vi "MALT132 get several output.vi"() -> ()   [LabVIEW 2018]
uses:
  <instrlib>/AltonTech MALT/AltonTech MALT200817.lvlib
panel:
  out "Status":u8[](array[numeric]) format="%02x"
  in  "Address":i32=3 format="%02x"
  in  "stop":bool
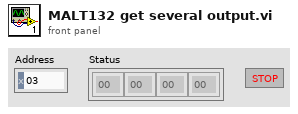
[diagram p1: front panel]
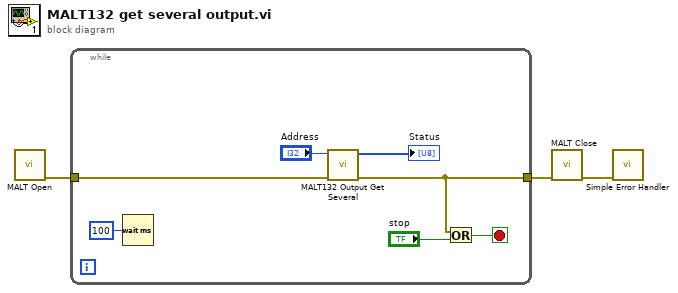
[diagram p0: block diagram]
diagram:
  n1 = call <instrlib>:"MALT Open.vi"() -> ("error out"=w3:errorcluster)  [unwired: 10 in, 1 out]
  n2 = while {
    tunnel: w3 -> [w10]
    tunnel: [w7] -> w2
    stop <- w5 stop-if-true
    n3 = Wait (ms)(milliseconds to wait=u32 100) -> ()  [unwired: 1 out]
    n4 = call <instrlib>:"MALT132 Output Get Several.vi"("error in"=w10, "Address"="Address") -> ("error out"=w7:errorcluster, "Status"=→"Status":u8[])  [unwired: 8 in]
    n5 = Or(x=w7, y="stop") -> (x .or. y?=w5:bool)
  }
  n6 = call <instrlib>:"MALT Close.vi"("error in"=w2) -> ("error out"=w1:errorcluster)  [unwired: 10 in]
  n7 = call <vilib>:"Simple Error Handler.vi"("error in (no error)"=w1) -> ()  [unwired: 4 in, 5 out]
